vi "MA2.vi"(0 "HWSerialNum":i32=83811664) -> (1 "MG17Motor 2":refnum<k7>, 2 "error out":errorcluster)   [LabVIEW 2014]
doc: "André Romero - 2016\nandretec@ifsc.usp.br\nIFSC - USP"
panel:
  in  "MG17Motor":refnum<k7>(container)
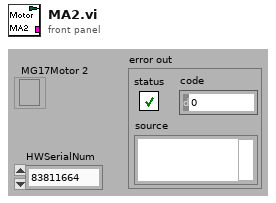
[diagram p1: front panel]
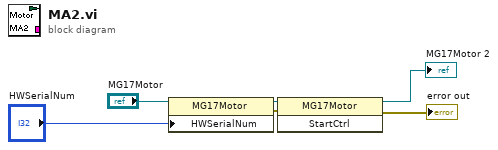
[diagram p0: block diagram]
diagram:
  n1 = property class="MG17Motor"(reference="MG17Motor", "HWSerialNum"="HWSerialNum") -> (reference out=w2:refnum<k7>, error out=w3:errorcluster)  [unwired: 1 in]
  n2 = invoke class="MG17Motor" method="StartCtrl"(reference=w2, error in=w3) -> (reference out=→"MG17Motor 2":refnum<k7>, error out=→"error out":errorcluster)  [unwired: 1 in, 1 out]
